vi "SaveSyringeConfiguration.vi"(0 "object in":refnum<class "CetoniPump.lvclass">, 2 "configuration file in":path, 4 "Write":T1(array[cluster]), 5 "error in (no error)":errorcluster) -> (14 "object out":refnum<class "CetoniPump.lvclass">, 19 "error out":errorcluster)   [LabVIEW 2021, in "CetoniPump.lvclass"]
uses:
  CetoniPump.lvclass
  <vilib>/Utility/config.llb/Write Key (Double).vi
  CetoniPump.lvclass/CetoniPump.ctl
  <vilib>/Utility/config.llb/NI_LVConfig.lvlib
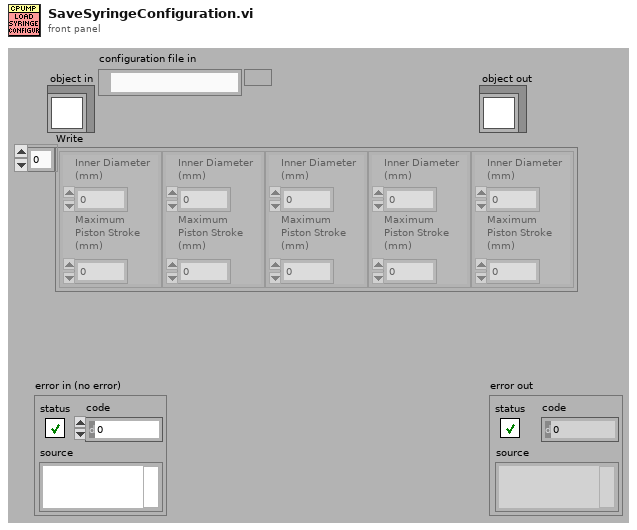
[diagram p1: front panel]
types:
  T1 = cluster{"Inner Diameter \n(mm)":dbl, "Maximum \nPiston Stroke \n(mm)":dbl}[]
  T2 = typedef "NI_LVConfig.lvlib/Config Data RefNum.ctl" = refnum<k1>
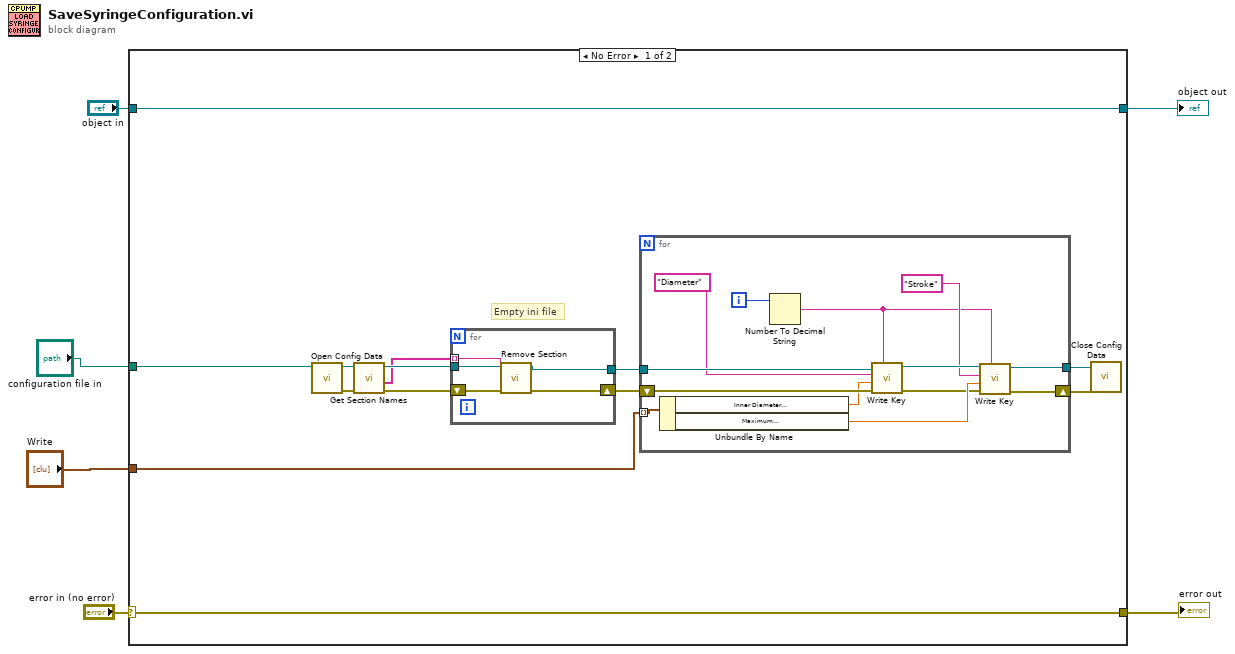
[diagram p0: block diagram]
diagram:
  n1 = case shown="No Error" "error in (no error)" {
    selector: "error in (no error)" -> [w19 w39]
    tunnel: [w19 w39] -> w5
    tunnel: [w18 w38] -> w3
    tunnel: "object in" -> [w18 w38]
    tunnel: "configuration file in" -> [w8 _]
    tunnel: "Write" -> [w7 _]
    frame No Error {
      # "Empty ini file"
      n2 = call <vilib>:"Open Config Data.vi"("configuration file path"=w8) -> ("error out"=w11:errorcluster, "refnum"=w17:T2)  [unwired: 8 in, 1 out]
      n3 = call <vilib>:"Get Section Names.vi"("error in (no error)"=w11, "refnum"=w17) -> ("error out"=w14:errorcluster, "section names"=w15:string[], "refnum out"=w16:T2)  [unwired: 7 in]
      n4 = for {
        tunnel: w16 -> [w37]
        tunnel: w15 -> [w36] mode=indexing
        tunnel: [w33] -> w12
        shift-right: [w34] -> w13
        shift-left: w14 -> [w35]
        n5 = call <vilib>:"Remove Section.vi"("section"=w36, "error in (no error)"=w35, "refnum"=w37) -> ("error out"=w34:errorcluster, "refnum out"=w33:T2)  [unwired: 6 in, 1 out]
      }
      n6 = for {
        tunnel: w12 -> [w31]
        tunnel: w7 -> [w27] mode=indexing
        tunnel: [w22] -> w10
        shift-right: [w21] -> w9
        shift-left: w13 -> [w32]
        i -> [w24]
        n7 = Unbundle By Name(w27) -> ("Inner Diameter \n(mm)"=w26:dbl, "Maximum \nPiston Stroke \n(mm)"=w25:dbl)
        n8 = Number To Decimal String(number=w24) -> (decimal integer string=w23:string)  [unwired: 1 in]
        n9 = call-poly <vilib>:"Write Key.vi"("section"=w23, "error in (no error)"=w32, "value"=w26, "key"="Diameter", "refnum"=w31) -> ("error out"=w20:errorcluster, "refnum out"=w30:T2)  [unwired: 4 in, 1 out]
        n10 = call-poly <vilib>:"Write Key.vi"("section"=w23, "error in (no error)"=w20, "value"=w25, "key"="Stroke", "refnum"=w30) -> ("error out"=w21:errorcluster, "refnum out"=w22:T2)  [unwired: 4 in, 1 out]
      }
      n11 = call <vilib>:"Close Config Data.vi"("error in (no error)"=w9, "refnum"=w10) -> ()  [unwired: 8 in, 2 out]
    }
    frame Error {
    }
  }
  "error out" <- w5
  "object out" <- w3
